vi "PlatformOffset.vi"(9 "Presets":T1, 10 "Buttons":bool[](array[boolean]), 11 "Lights Values":T2) -> (2 "offset":enum16{"Step", "platform", "Ground"}(ring))   [LabVIEW 2014]
doc: "Set the new ground offset if a button is pressed. Light up the correct button"
uses:
  LEDdriver/LEDPorts.ctl
  buttons/PresetValues.ctl
  <vilib>/Rock Robotics/Network Tables/SD Read Number.vi
  <vilib>/Rock Robotics/Network Tables/SD Write Boolean.vi
  <vilib>/Rock Robotics/Network Tables/SD Write Number.vi
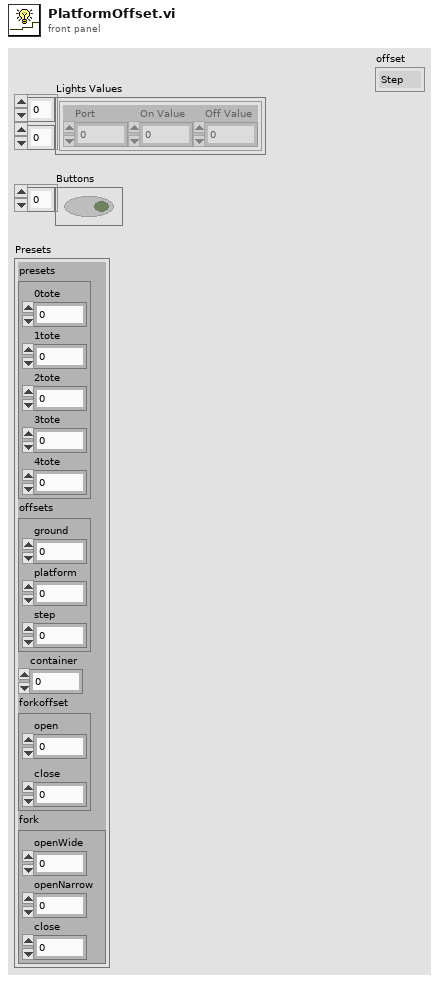
[diagram p1: front panel]
types:
  T1 = typedef "PresetValues.ctl" = cluster{"presets":cluster{"0tote":dbl, "1tote":dbl, "2tote":dbl, "3tote":dbl, "4tote":dbl}, "offsets":cluster{"ground":dbl, "platform":dbl, "step":dbl}, "container":dbl, "forkoffset":cluster{"open":dbl, "close":dbl}, "fork":cluster{"openWide":dbl, "openNarrow":dbl, "close":dbl}}
  T2 = typedef "LEDPorts.ctl" = cluster{"Port":i16, "On Value":u8, "Off Value":u8}[][]
  T3 = cluster{"ground":dbl, "platform":dbl, "step":dbl}
  T4 = cluster{"Port":i16, "On Value":u8, "Off Value":u8}
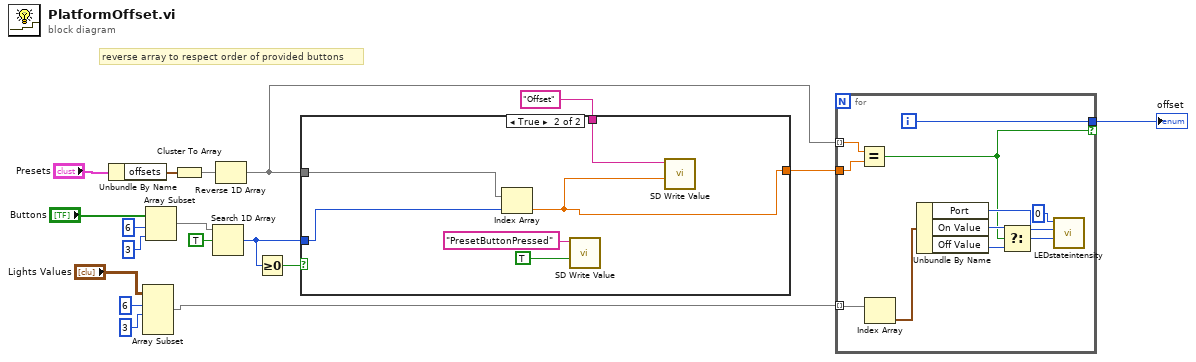
[diagram p0: block diagram]
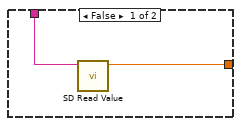
[diagram p2: hidden frame]
diagram:
  # "reverse array to respect order of provided buttons"
  n1 = Unbundle By Name("Presets") -> ("offsets"=w9:T3)
  n2 = Array Subset(array="Lights Values", index (row)=6 ("index"), length (row)=3 ("length")) -> (w2:T2)  [unwired: 2 in]
  n3 = Array Subset(array="Buttons", index=6, length=3) -> (w15:bool[])
  n4 = Cluster To Array(cluster=w9) -> (array=w10:dbl[])
  n5 = Search 1D Array(1D array=w15, element=TRUE) -> (index of element=w12:i32)  [unwired: 1 in]
  n6 = Reverse 1D Array(array=w10) -> (reversed array=w7:dbl[])
  n7 = Greater Or Equal To 0?(x=w12) -> (x >= 0?=w13:bool)
  n8 = case shown="True" w13 {
    tunnel: w12 -> [_ w26]
    tunnel: "Offset" ("Name") -> [w20 w25]
    tunnel: [w19 w24] -> w6
    tunnel: w7 -> [_ w23]
    frame False {
      n9 = call-poly <vilib>:"SD Read Value.vi"("Name"=w20) -> ("Numeric"=w19:dbl)  [unwired: 8 in, 2 out]
    }
    frame True {
      n10 = Index Array(array=w23, index=w26) -> (element=w24:dbl)
      n11 = call-poly <vilib>:"SD Write Value.vi"("Boolean"=TRUE, "Name"="PresetButtonPressed") -> ()  [unwired: 8 in, 2 out]
      n12 = call-poly <vilib>:"SD Write Value.vi"("Numeric"=w24, "Name"=w25) -> ()  [unwired: 8 in, 2 out]
    }
  }
  n13 = for {
    tunnel: w7 -> [w35] mode=indexing
    tunnel: w6 -> [w36]
    tunnel: w2 -> [w37] mode=indexing
    tunnel: [w28] -> w1 if=w27
    i -> [w28]
    n14 = Equal?(x=w35, y=w36) -> (x = y?=w27:bool)
    n15 = Index Array(array=w37) -> (element=w34:T4)  [unwired: 1 in]
    n16 = Unbundle By Name(w34) -> ("Port"=w30:i16, "On Value"=w33:u8, "Off Value"=w32:u8)
    n17 = Select(t=w33, s=w27, f=w32) -> (s? t:f=w31:u8)
    n18 = call "LEDstateintensity.vi"("intensity"=w31, "port"=w30, "Id"=i16 0) -> ()  [unwired: 6 in, 3 out]
  }
  "offset" <- w1
